vi "Core.vi"(0 "VI Reference In":refnum<vi>, 1 "Label":string, 2 "delimiter (>>)":string=">>", 3 "Assert Only? (F)":bool, 5 "Control Name":string, 7 "Disabled":T1(ring), 11 "Error In":errorcluster, 12 "Assert Interval(10 ms)":u32=10, 13 "Timeout(5 sec)":dbl=5.0) -> (4 "VI Reference Out":refnum<vi>, 15 "Error Out":errorcluster)   [LabVIEW 2016, in "Drona.lvlib" / "AssertControlDisable.lvlib"]
doc: "Asserts the state of controls.\n\nThe input control name is given as a string , incase of path, use delimiters inbetween the path."
uses:
  AssertControlDisable.lvlib
  Setup/GetControlRef/GetControlRefByPath.vi
  <vilib>/addons/_JKI Toolkits/Caraya/classes/Assert/Assert Equal Value and Type_Variant.vi
  <vilib>/addons/_JKI Toolkits/Caraya/classes/Assert/Assert.lvclass
  Setup/GetControlRef/GetControlRef.lvlib
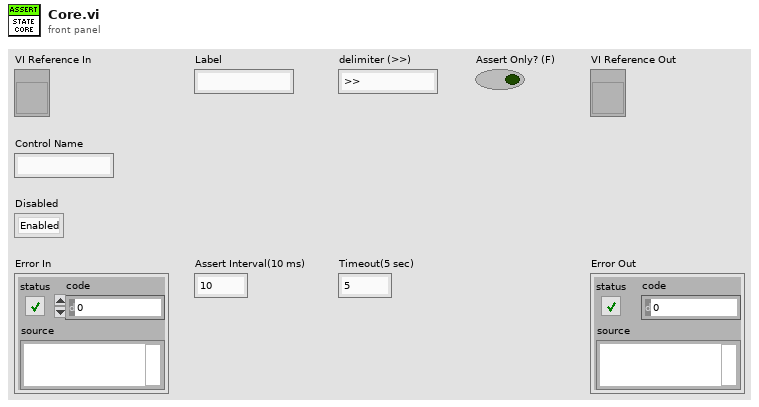
[diagram p1: front panel]
types:
  T1 = enum8{"Enabled", "Disabled", "Disabled and Grayed Out"}
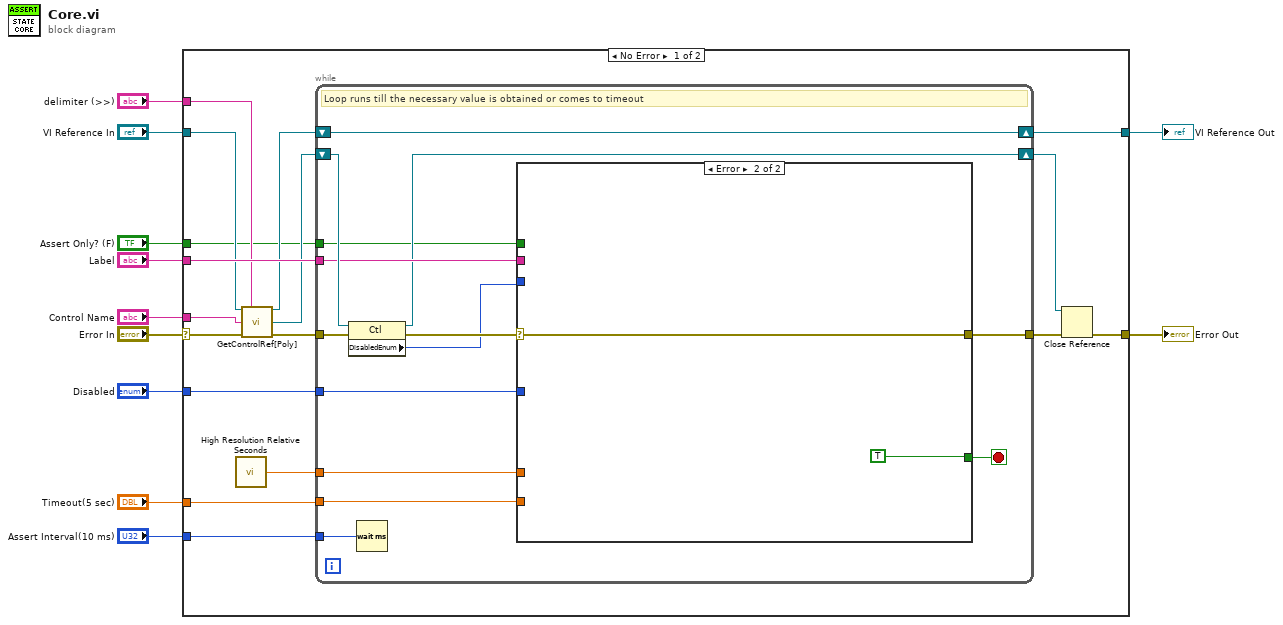
[diagram p0: block diagram]
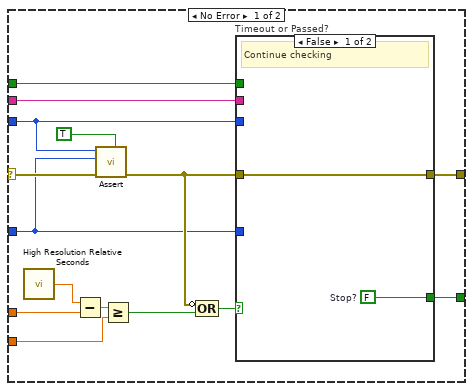
[diagram p2: hidden frame]
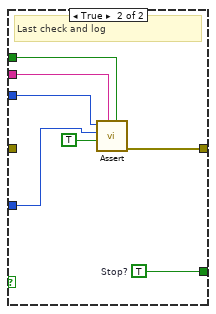
[diagram p3: hidden frame]
diagram:
  n1 = case shown="No Error" "Error In" {
    selector: "Error In" -> [w23 w70]
    tunnel: "Timeout(5 sec)" -> [w28 _]
    tunnel: [w27 w69] -> w10
    tunnel: [w16 w70] -> w9
    tunnel: "Assert Interval(10 ms)" -> [w25 _]
    tunnel: "Label" -> [w24 _]
    tunnel: "VI Reference In" -> [w22 w69]
    tunnel: "Control Name" -> [w21 _]
    tunnel: "delimiter (>>)" -> [w14 _]
    tunnel: "Assert Only? (F)" -> [w13 _]
    tunnel: "Disabled" -> [w12 _]
    frame No Error {
      n2 = call <vilib>:"High Resolution Relative Seconds.vi"() -> ("relative seconds"=w20:dbl)
      n3 = call-poly "GetControlRef[Poly].vi"("VI Reference In"=w22, "delimiter (>>)"=w14, "Control Name"=w21, "error In"=w23) -> ("VI Reference Out"=w18:refnum<vi>, "Ctl Refnum"=w17:refnum<vi>, "error out"=w19:errorcluster)  [unwired: 9 in]
      n4 = while {
        tunnel: w28 -> [w41]
        tunnel: w20 -> [w42]
        tunnel: w19 -> [w36]
        tunnel: [w39] -> w26
        tunnel: w25 -> [w37]
        tunnel: w24 -> [w33]
        shift-right: [w34] -> w27
        shift-left: w18 -> [w34]
        shift-right: [w32] -> w15
        shift-left: w17 -> [w35]
        tunnel: w13 -> [w31]
        tunnel: w12 -> [w29]
        stop <- w40 stop-if-true
        # "Loop runs till the necessary value is obtained or comes to timeout"
        n5 = property class="Ctl"(reference=w35, error in=w36) -> (reference out=w32:refnum<vi>, error out=w38:errorcluster, "DisabledEnum"=w30:T1)
        n6 = Wait (ms)(milliseconds to wait=w37) -> ()  [unwired: 1 out]
        n7 = case shown="Error" w38 {
          selector: w38 -> [w53 w68]
          tunnel: w42 -> [w57 _]
          tunnel: w41 -> [w54 _]
          tunnel: [w46 TRUE] -> w40
          tunnel: [w47 w68] -> w39
          tunnel: w30 -> [w45 _]
          tunnel: w33 -> [w52 _]
          tunnel: w31 -> [w44 _]
          tunnel: w29 -> [w43 _]
          frame No Error {
            n8 = call <vilib>:"High Resolution Relative Seconds.vi"() -> ("relative seconds"=w56:dbl)
            n9 = Subtract(x=w56, y=w57) -> (x-y=w55:dbl)
            n10 = call-poly <vilib>:"Assert.vi"("Assert Only? (F)"=TRUE, "error in (no error)"=w53, "Y"=w43, "X"=w45) -> ("error out"=w50:errorcluster)  [unwired: 7 in]
            n11 = Greater Or Equal?(x=w55, y=w54) -> (x >= y?=w51:bool)
            n12 = Compound Arithmetic op=OR(invert w50, w51) -> (w49:bool)
            n13 = case "Timeout or Passed?" shown="False" w49 {
              tunnel: w50 -> [w59 _]
              tunnel: w45 -> [_ w65]
              tunnel: w52 -> [_ w66]
              tunnel: [w59 w64] -> w47
              tunnel: [w58 w63] -> w46
              tunnel: w44 -> [_ w61]
              tunnel: w43 -> [_ w60]
              frame False {
                w58 = FALSE  # Stop?
                # "Continue checking"
              }
              frame True {
                w63 = TRUE  # Stop?
                # "Last check and log"
                n14 = call-poly <vilib>:"Assert.vi"("Assert Only? (F)"=w61, "Label"=w66, "Register with caller test (F)"=TRUE, "Y"=w60, "X"=w65) -> ("error out"=w64:errorcluster)  [unwired: 6 in]
              }
            }
          }
          frame Error {
          }
        }
      }
      n15 = Close Reference(reference=w15, error in (no error)=w26) -> (error out=w16:errorcluster)
    }
    frame Error {
    }
  }
  "Error Out" <- w9
  "VI Reference Out" <- w10
